vi "Remove State Connection.vi"(8 "error in (no error)":errorcluster, 9 "Connection":T1, 10 "State":string, 11 "Channel Ref in":T2 format="%.0x") -> (0 "error out":errorcluster, 3 "Channel Ref out":T2=18446744073709551615 format="%.0x")   [LabVIEW 2017, in "Routing and Faulting Scripting.lvlib"]
uses:
  Routing and Faulting Scripting.lvlib
  <vilib>/NI Veristand/Custom Device API/Custom Device Item Ref.ctl
  Shared/Connection.ctl
  NationalInstruments.VeriStand.SystemDefinitionAPI
  Constants/Scripting Constants.vi
  <vilib>/NI Veristand/Custom Device API/Custom Device API.lvlib
  Shared/Routing and Faulting Shared.lvlib
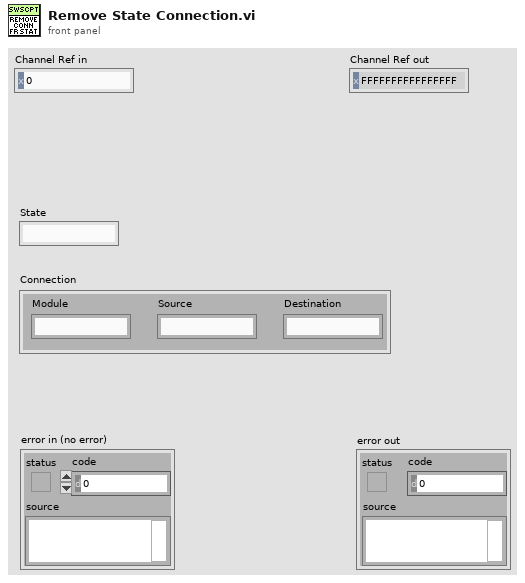
[diagram p1: front panel]
types:
  T1 = typedef "Routing and Faulting Shared.lvlib/Connection.ctl" = cluster{"Module":string, "Source":string, "Destination":string}
  T2 = typedef "Custom Device API.lvlib/Custom Device Item Ref.ctl" = u64
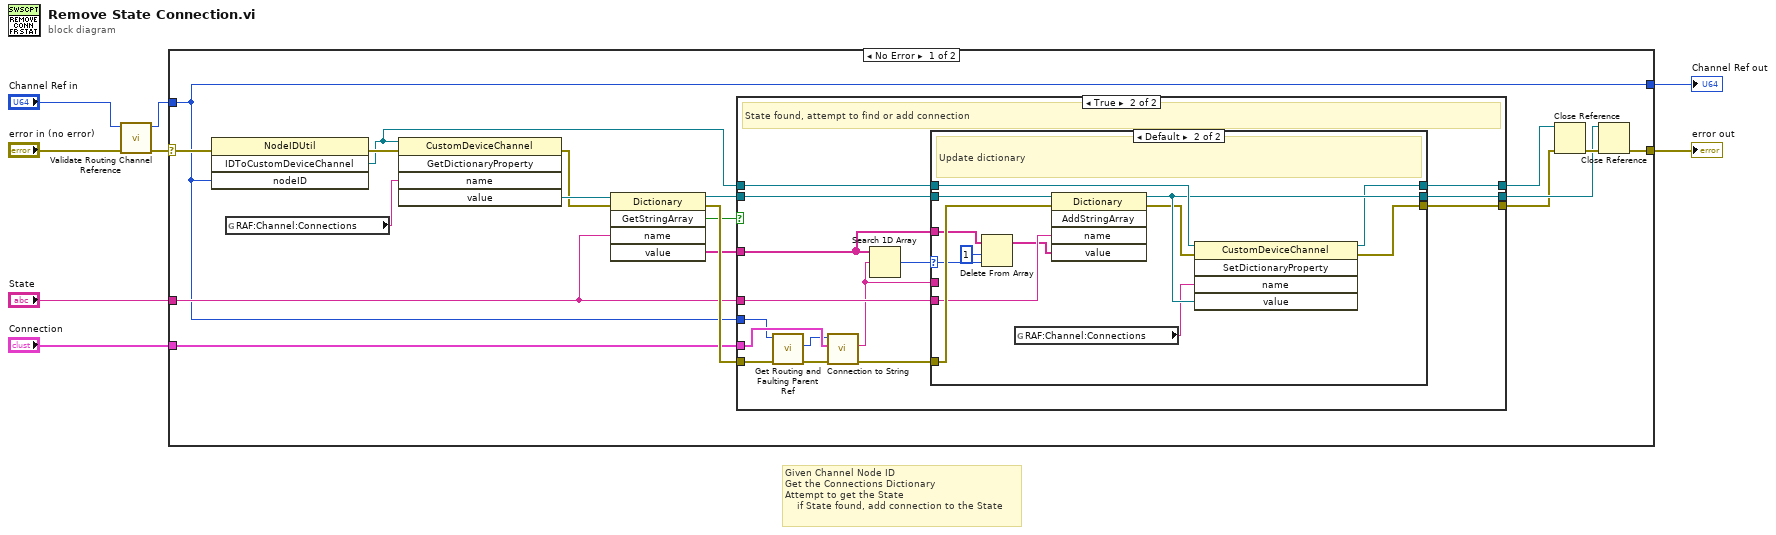
[diagram p0: block diagram]
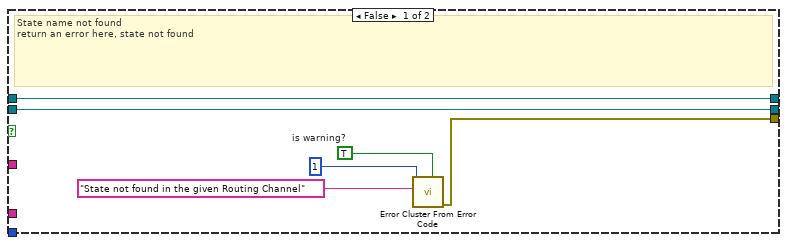
[diagram p2: hidden frame]
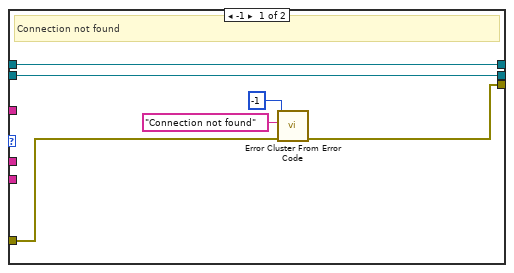
[diagram p3: hidden frame]
diagram:
  # "Given Channel Node ID\nGet the Connections Dictionary\nAttempt to get the State\n    if State found, add connection to the State"
  n1 = call "Validate Routing Channel Reference.vi"("error in (no error)"="error in (no error)", "Channel Ref in"="Channel Ref in") -> ("error out"=w3:errorcluster, "Channel Ref out"=w1:T2)  [unwired: 8 in]
  n2 = case shown="No Error" w3 {
    selector: w3 -> [w22 w68]
    tunnel: [w25 w68] -> w7
    tunnel: w1 -> [w9 w67]
    tunnel: [w9 w67] -> w6
    tunnel: "State" -> [w16 _]
    tunnel: "Connection" -> [w11 _]
    frame No Error {
      n3 = invoke class="NodeIDUtil" method="IDToCustomDeviceChannel"(error in=w22, "nodeID"=w9) -> (error out=w23:errorcluster, "IDToCustomDeviceChannel"=w13:refnum<k24>)  [unwired: 2 in, 2 out]
      n4 = global read "Scripting Constants.vi" "RAF:Channel:Connections"() -> (w10:string)
      n5 = invoke class="CustomDeviceChannel" method="GetDictionaryProperty"(reference=w13, error in=w23, "name"=w10) -> (error out=w19:errorcluster, "value"=w20:refnum<k24>)  [unwired: 2 in, 3 out]
      n6 = invoke class="Dictionary" method="GetStringArray"(reference=w20, error in=w19, "name"=w16) -> (reference out=w17:refnum<k24>, error out=w26:errorcluster, "GetStringArray"=w18:bool, "value"=w21:string[])  [unwired: 2 in, 1 out]
      n7 = case shown="True" w18 {
        tunnel: w21 -> [_ w40]
        tunnel: w26 -> [_ w36]
        tunnel: [w29 w46] -> w14
        tunnel: w16 -> [_ w45]
        tunnel: w17 -> [w28 w44]
        tunnel: [w28 w43] -> w15
        tunnel: w13 -> [w27 w42]
        tunnel: [w27 w41] -> w12
        tunnel: w11 -> [_ w39]
        tunnel: w9 -> [_ w33]
        frame False {
          w31 = TRUE  # is warning?
          # "State name not found\nreturn an error here, state not found"
          n8 = call <vilib>:"Error Cluster From Error Code.vi"("is warning? (False)"=w31, "error message (\"\")"="State not found in the given Routing Channel" ("error message (\"\")"), "error code (0)"=1) -> ("error out"=w29:errorcluster)  [unwired: 6 in]
        }
        frame True {
          # "State found, attempt to find or add connection"
          n9 = call "Get Routing and Faulting Parent Ref.vi"("error in (no error)"=w36, "Routing and Faulting Child Ref in"=w33) -> ("error out"=w35:errorcluster, "Routing and Faulting Ref out"=w34:T2)  [unwired: 7 in, 1 out]
          n10 = call "Connection to String.vi"("error in (no error)"=w35, "Connection"=w39, "Routing and Faulting Ref in"=w34) -> ("error out"=w37:errorcluster, "String"=w38:string)  [unwired: 6 in, 1 out]
          n11 = Search 1D Array(1D array=w40, element=w38) -> (index of element=w47:i32)  [unwired: 1 in]
          n12 = case shown="Default" w47 {
            selector: w47 -> [_ w57]
            tunnel: w37 -> [w51 w66]
            tunnel: [w50 w60] -> w46
            tunnel: w45 -> [_ w65]
            tunnel: w44 -> [w49 w64]
            tunnel: [w49 w62] -> w43
            tunnel: w42 -> [w48 w63]
            tunnel: [w48 w59] -> w41
            tunnel: w40 -> [_ w58]
            tunnel: w38 -> [_ _]
            frame -1 {
              # "Connection not found"
              n13 = call <vilib>:"Error Cluster From Error Code.vi"("error in (no error)"=w51, "error message (\"\")"="Connection not found" ("error message (\"\")"), "error code (0)"=-1) -> ("error out"=w50:errorcluster)  [unwired: 6 in]
            }
            frame Default {
              # "Update dictionary"
              n14 = Delete From Array(array=w58, length=1, index=w57) -> (array with subset deleted=w56:string[])  [unwired: 1 out]
              n15 = global read "Scripting Constants.vi" "RAF:Channel:Connections"() -> (w54:string)
              n16 = invoke class="Dictionary" method="AddStringArray"(reference=w64, error in=w66, "name"=w65, "value"=w56) -> (reference out=w62:refnum<k24>, error out=w61:errorcluster)  [unwired: 1 in, 3 out]
              n17 = invoke class="CustomDeviceChannel" method="SetDictionaryProperty"(reference=w63, error in=w61, "name"=w54, "value"=w62) -> (reference out=w59:refnum<k24>, error out=w60:errorcluster)  [unwired: 1 in, 3 out]
            }
          }
        }
      }
      n18 = Close Reference(reference=w12, error in (no error)=w14) -> (error out=w24:errorcluster)
      n19 = Close Reference(reference=w15, error in (no error)=w24) -> (error out=w25:errorcluster)
    }
    frame Error {
    }
  }
  "Channel Ref out" <- w6
  "error out" <- w7
